vi "Flatten PDU.vi"(8 "error in":errorcluster, 11 "ELAN data unit in":refnum<class "ELAN PDU.lvclass">) -> (0 "error out":errorcluster, 3 "Full ELAN data unit":u8[](array[numeric]) format="%x")   [LabVIEW 2021, in "ELAN PDU.lvclass"]
uses:
  ELAN PDU.lvclass
  ELAN PDU.lvclass/ELAN PDU.ctl
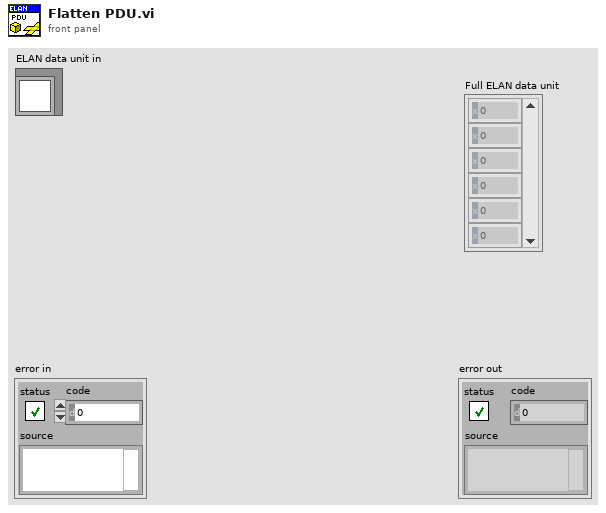
[diagram p1: front panel]
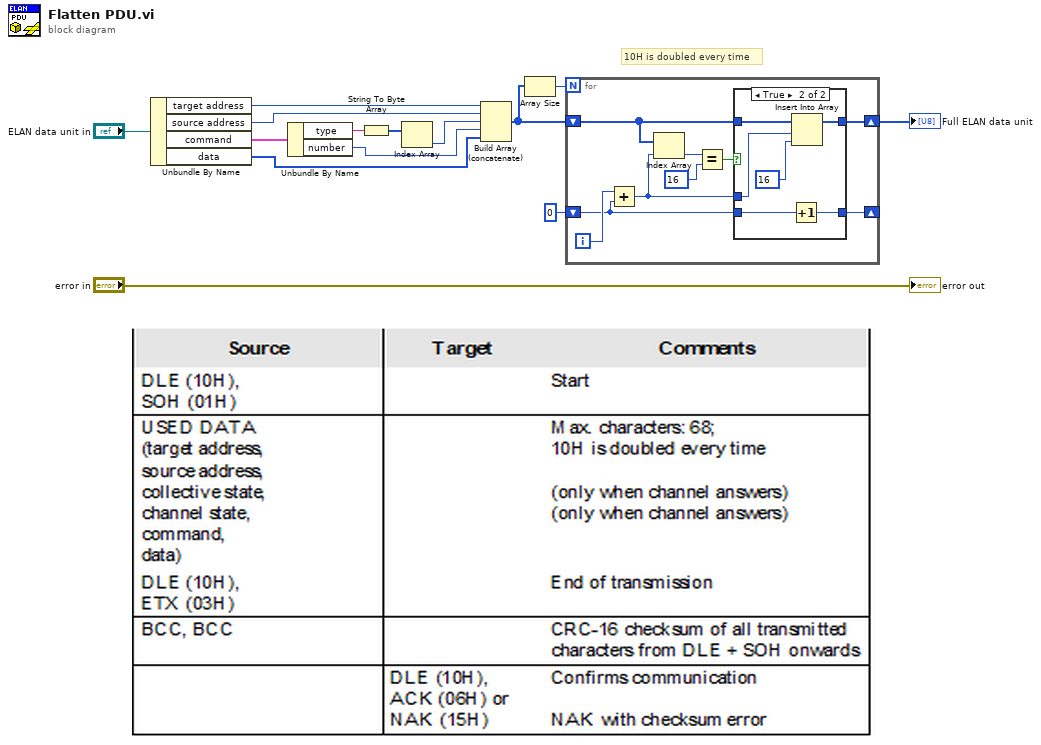
[diagram p0: block diagram]
diagram:
  # "10H is doubled every time"
  n1 = Unbundle By Name("ELAN data unit in") -> ("target address"=w9:u8, "source address"=w8:u8, "command"=w12:cluster{"type":string, "number":u8}, "data"=w5:u8[])
  n2 = Unbundle By Name(w12) -> ("type"=w11:string, "number"=w6:u8)
  n3 = String To Byte Array(string=w11) -> (unsigned byte array=w10:u8[])
  n4 = Index Array(array=w10) -> (element=w7:u8)  [unwired: 1 in]
  n5 = Build Array (concatenate)(w9, w8, w7, w6, w5) -> (w2:u8[])
  n6 = Array Size(array=w2) -> (size(s)=w3:i32)
  n7 = for {
    N: w3 -> [_]
    shift-right: [w19] -> w4
    shift-left: w2 -> [w22]
    shift-right: [w18] -> _
    shift-left: 0 -> [w15]
    i -> [w16]
    n8 = Add(x=w16, y=w15) -> (x+y=w17:i32)
    n9 = Index Array(array=w22, index=w17) -> (element=w23:u8)
    n10 = Equal?(x=w23, y=u8 16) -> (x = y?=w20:bool)
    n11 = case shown="True" w20 {
      tunnel: w22 -> [w25 w31]
      tunnel: w17 -> [_ w28]
      tunnel: [w25 w29] -> w19
      tunnel: [w24 w27] -> w18
      tunnel: w15 -> [w24 w26]
      frame False {
      }
      frame True {
        n12 = Increment(x=w26) -> (x+1=w27:i32)
        n13 = Insert Into Array(array=w31, index=w28, new element=u8 16 ("y")) -> (w29:u8[])
      }
    }
  }
  "Full ELAN data unit" <- w4
  "error out" <- "error in"
